vi "Error.vi"(8 "Error In":errorcluster, 11 "object in":refnum<class "Connected.lvclass">) -> (0 "Error Out":errorcluster, 3 "FGEN States":refnum<class "IStates.lvclass">)   [LabVIEW 2023, in "HAL.lvlib" / "PXI-5441.lvlib" / "Connected.lvclass"]
uses:
  Connected.lvclass
  FGEN_class/states/IStates_interface/IStates.lvclass
  Error_class/Error.lvclass
  Connected.lvclass/Connected.ctl
  D:/git/HAL/PXI-5441_class/states/Error_class/Error.lvclass
  D:/git/HAL/FGEN_class/states/IStates_interface/IStates.lvclass
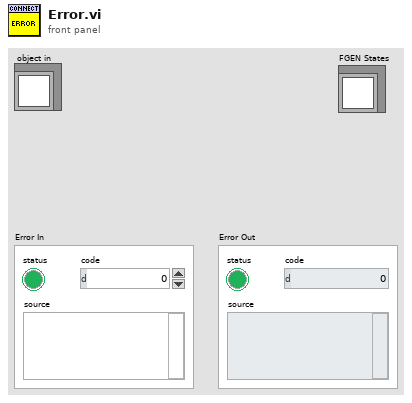
[diagram p1: front panel]
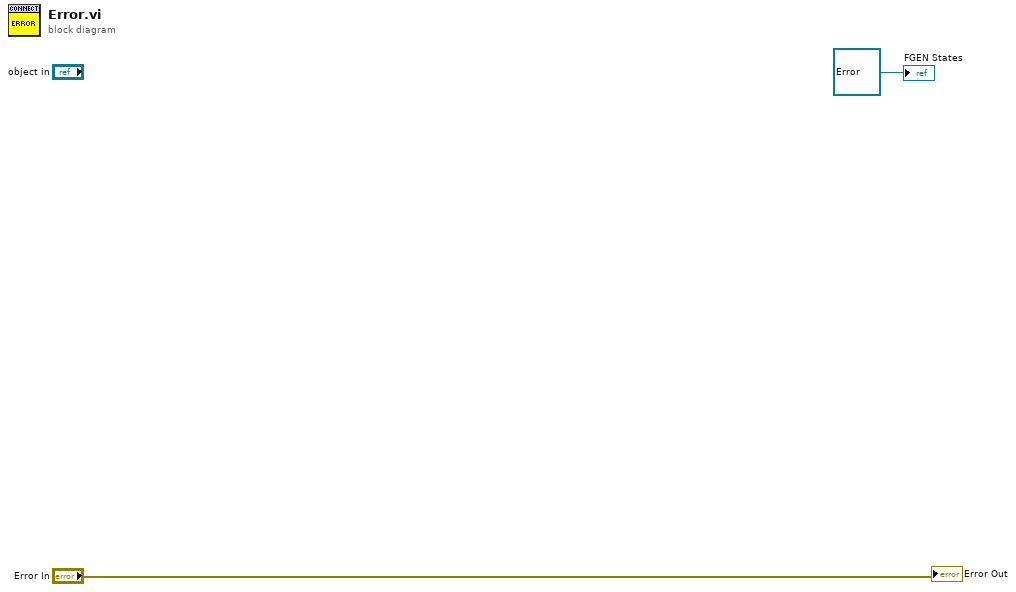
[diagram p0: block diagram]
diagram:
  "Error Out" <- "Error In"
  "FGEN States" <- refnum<class "Error.lvclass"> refnum ("PXI-5441.lvlib:Error")
